vi "xPCScGetData.vi"(1 "numsamples":i32, 4 "buffer":dbl[](array[numeric]) format="%.26e", 5 "start":i32, 6 "error in (no error)":errorcluster, 7 "signal_id":i32, 8 "decimation":i32, 9 "scope":i32, 10 "port":i32) -> (0 "error out":errorcluster, 2 "data":dbl[](array[numeric]) format="%.26e", 3 "port copy":i32)   [LabVIEW 2018]
uses:
  XPCAPI.DLL
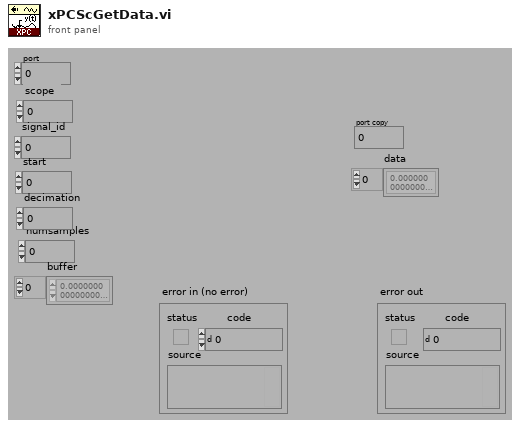
[diagram p1: front panel]
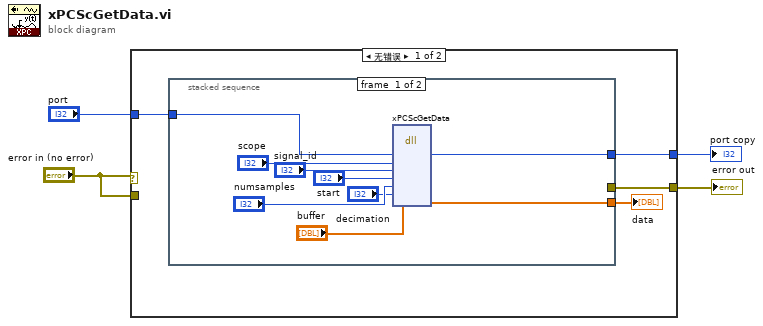
[diagram p0: block diagram]
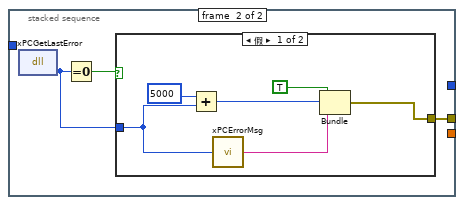
[diagram p2: hidden frame]
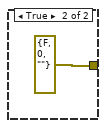
[diagram p3: hidden frame]
diagram:
  n1 = case shown="无错误" "error in (no error)" {
    tunnel: [w8 w29] -> w4
    tunnel: "error in (no error)" -> [_ w29]
    tunnel: "port" -> [w7 w28]
    tunnel: [w6 w28] -> w1
    frame No Error {
      n2 = stacked-sequence {
        tunnel: [w11 _] -> w6
        tunnel: [_ w18] -> w8
        tunnel: w7 -> [w10 _]
        tunnel: [w9 _] -> w5
        frame #0 {
          n3 = dll-call lib="PTH2Iabs CUsers\nyuchengxinDesktop上下位机联机测试\nxpcapi.dll" fn="xPCScGetData"("port"=w10, "scope"="scope", "signal_id"="signal_id", "start"="start", "numsamples"="numsamples", "decimation"="decimation", "data"="buffer") -> ("port"=w11:i32, "data"=w9:dbl[])  [unwired: 9 in, 2 out]
        }
        frame #1 {
          n4 = dll-call lib="PTH2Iabs CUsers\nyuchengxinDesktop上下位机联机测试\nxpcapi.dll" fn="xPCGetLastError"() -> (w19:i32)  [unwired: 3 in, 2 out]
          n5 = Equal To 0?(x=w19) -> (x = 0?=w20:bool)
          n6 = case shown="假" w20 {
            tunnel: w19 -> [w22 _]
            tunnel: [w23 errorcluster {"status"=FALSE, "code"=0, "source"=""} ("error out")] -> w18
            frame False {
              n7 = Add(x=5000 ("y"), y=w22) -> (x+y=w25:i32)
              n8 = call "xPCErrorMsg.vi"("error number"=w22) -> ("ErrorMsg"=w24:string)
              n9 = Bundle(TRUE, w25, "ErrorMsg"=w24) -> (w23:cluster{bool, i32, "ErrorMsg":string})  [unwired: 1 in]
            }
            frame True {
            }
          }
        }
      }
      "data" <- w5
    }
    frame Error {
    }
  }
  "port copy" <- w1
  "error out" <- w4
